vi "Update Status String.vi"(8 "error in (no error)":errorcluster, 10 "Append this string":string, 11 "object in":refnum<class "Tesla Factory Tester.lvclass">) -> (0 "error out":errorcluster, 3 "object out":refnum<class "Tesla Factory Tester.lvclass">)   [LabVIEW 2013, in "Tesla Factory Tester.lvlib" / "Tesla Factory Tester.lvclass"]
uses:
  Tesla Factory Tester.lvclass
  Tesla Factory Tester.lvclass/Tesla Factory Tester.ctl
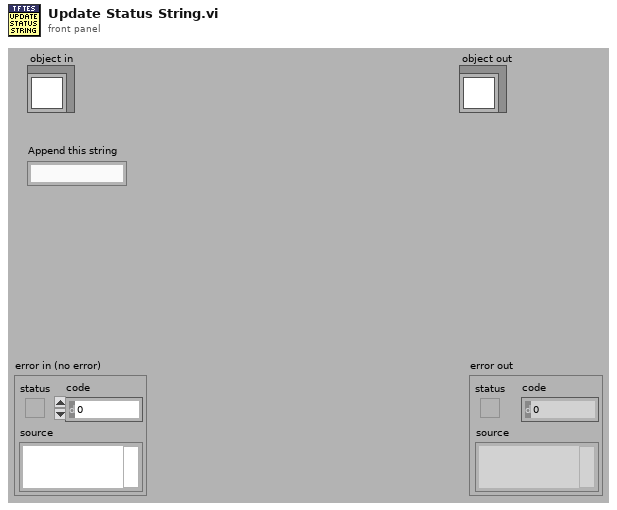
[diagram p1: front panel]
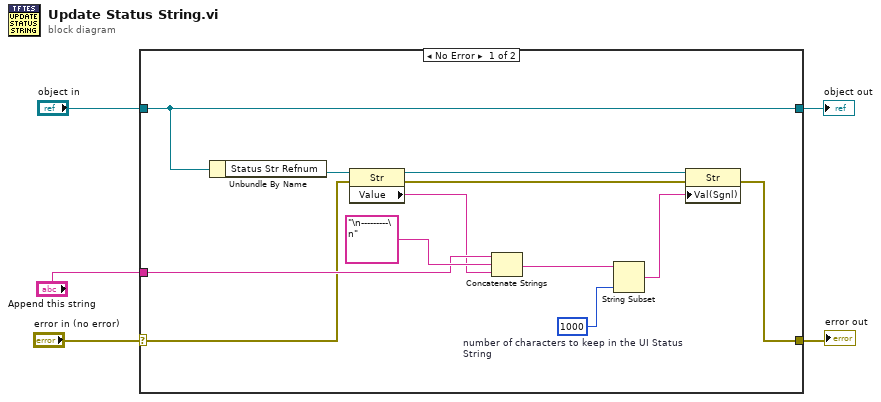
[diagram p0: block diagram]
diagram:
  n1 = case shown="No Error" "error in (no error)" {
    selector: "error in (no error)" -> [w11 w19]
    tunnel: [w6 w19] -> w4
    tunnel: [w17 w18] -> w2
    tunnel: "object in" -> [w17 w18]
    tunnel: "Append this string" -> [w13 _]
    frame No Error {
      w14 = 1000  # number of characters to keep in the UI Status String
      n2 = Unbundle By Name(w17) -> ("Status Str Refnum"=w16:refnum<vi>)
      n3 = property class="Str"(reference=w16, error in=w11) -> (reference out=w9:refnum<vi>, error out=w8:errorcluster, "Value"=w12:string)
      n4 = Concatenate Strings(w13, "\n---------\n" ("string"), w12) -> (w10:string)
      n5 = String Subset(string=w10, length (rest)=w14) -> (substring=w7:string)  [unwired: 1 in]
      n6 = property class="Str"(reference=w9, error in=w8, "Val(Sgnl)"=w7) -> (error out=w6:errorcluster)  [unwired: 1 out]
    }
    frame Error {
    }
  }
  "error out" <- w4
  "object out" <- w2
